vi "ObjectHandler.ExitReference.vi"(8 "error in (no error)":errorcluster, 10 "Name":string, 11 "ObjectHandler in":refnum<class "ObjectHandler.lvclass">) -> (0 "error out":errorcluster, 3 "ObjectHandler out":refnum<class "ObjectHandler.lvclass">)   [LabVIEW 2016, in "ObjectHandler.lvclass"]
uses:
  ObjectHandler.lvclass
  ObjectHandler.ObjectWType.ctl
  ObjectHandler.ObjectType.ctl
  ObjectHandler.lvclass/ObjectHandler.ctl
  ViHandler/ViHandler.lvclass
  Package ErrorHandling/ErrorHandling.lvclass
  CentralStorage/CentralStorage.lvclass
  Package Simulation/Modell/Hausmodell/Hausmodell.lvclass
  Package Simulation/Modell/Sondenmodell/Sondenmodell.lvclass
  Package Simulation/Modell/Umgebung/Umgebung.lvclass
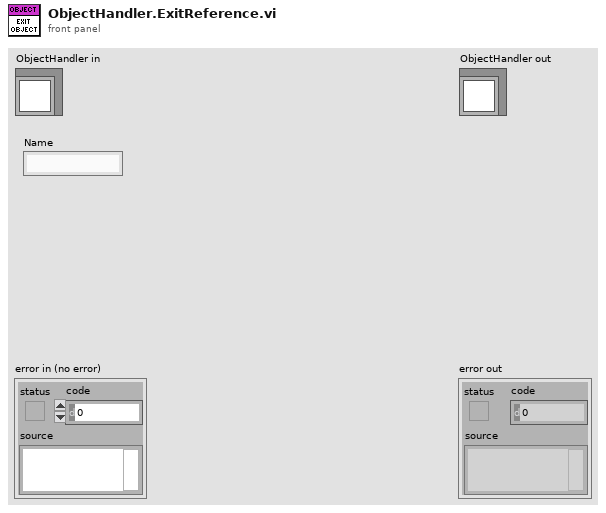
[diagram p1: front panel]
types:
  T1 = typedef "ObjectHandler.lvclass/ObjectHandler.ObjectWType.ctl" = cluster{"ObjectType":T2, "Object":variant}
  T2 = typedef "ObjectHandler.lvclass/ObjectHandler.ObjectType.ctl" = enum16{"undefined", "ObjectHandler", "ViHandler", "ErrorHandler", "CentralStorage", "Hausmodell", "Sondenmodell", "Wärmepumpe", "Umgebung"}
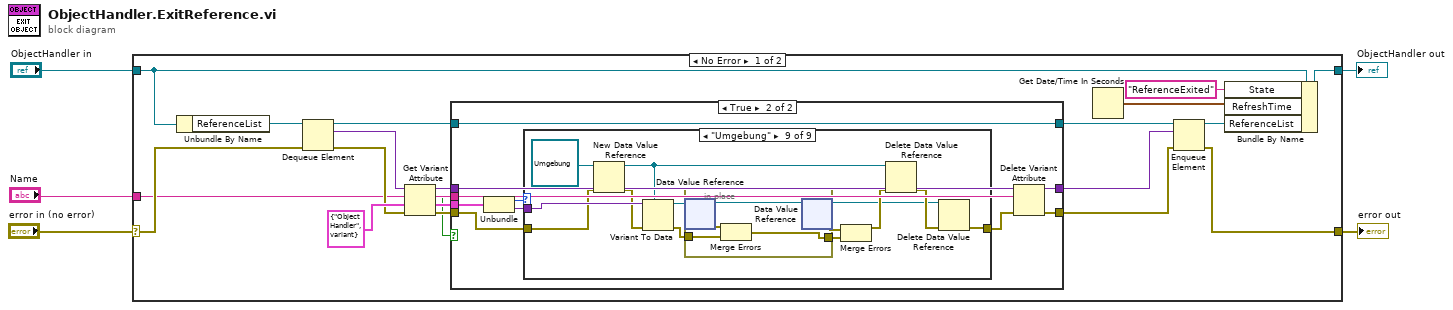
[diagram p0: block diagram]
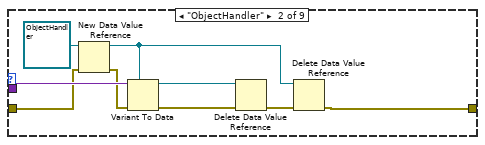
[diagram p4: hidden frame]
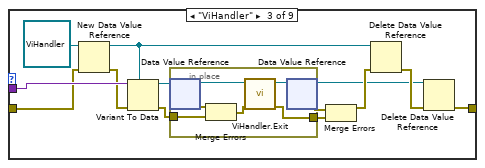
[diagram p5: hidden frame]
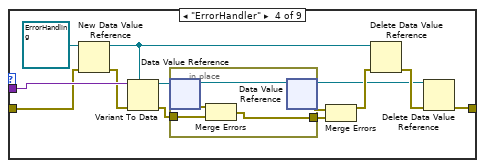
[diagram p6: hidden frame]
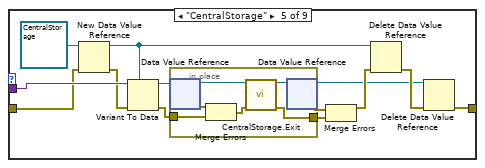
[diagram p7: hidden frame]
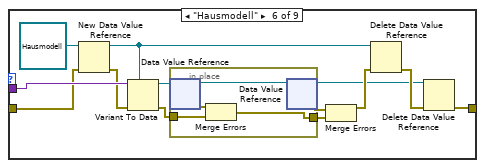
[diagram p8: hidden frame]
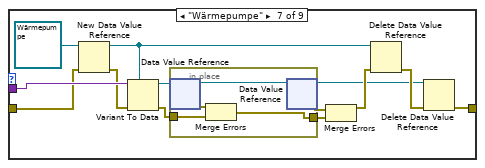
[diagram p9: hidden frame]
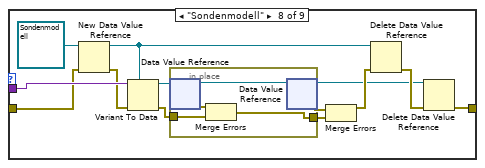
[diagram p10: hidden frame]
diagram:
  n1 = case shown="No Error" "error in (no error)" {
    selector: "error in (no error)" -> [w18 w173]
    tunnel: [w12 w173] -> w4
    tunnel: [w20 w172] -> w2
    tunnel: "ObjectHandler in" -> [w24 w172]
    tunnel: "Name" -> [w9 _]
    frame No Error {
      n2 = Unbundle By Name(w24) -> ("ReferenceList"=w19:refnum<queue>)
      n3 = Dequeue Element(queue=w19, error in (no error)=w18) -> (queue out=w7:refnum<queue>, element=w17:variant, error out=w16:errorcluster)  [unwired: 1 in, 1 out]
      n4 = Get Variant Attribute(Variant=w17, name=w9, default value (empty Variant)=T1 {"ObjectType"=enum."ObjectHandler", "Object"=variant} ("ObjectWType"), error in=w16) -> (duplicate Variant=w21:variant, found=w8:bool, value=w23:T1, error out=w22:errorcluster)
      n5 = case shown="True" w8 {
        tunnel: w23 -> [_ w36]
        tunnel: w22 -> [w28 w35]
        tunnel: w21 -> [w27 w33]
        tunnel: [w27 w32] -> w14
        tunnel: [w28 w31] -> w13
        tunnel: w9 -> [_ w30]
        tunnel: w7 -> [w26 w29]
        tunnel: [w26 w29] -> w6
        frame False {
        }
        frame True {
          n6 = Unbundle(w36) -> ("ObjectType"=w37:T2, "Object"=w38:variant)
          n7 = case shown="\"Umgebung\"" w37 {
            tunnel: w38 -> [_ w47 w61 w80 w97 w116 w133 w150 w167]
            tunnel: w35 -> [w39 w45 w59 w78 w95 w114 w131 w148 w165]
            tunnel: [w39 w40 w56 w75 w92 w111 w128 w145 w162] -> w34
            frame "undefined", Default {
            }
            frame "ObjectHandler" {
              n8 = New Data Value Reference(data value=refnum<class "ObjectHandler.lvclass"> refnum ("ObjectHandler.lvclass"), error in=w45) -> (data value reference=w44:refnum<data-value>, error out=w46:errorcluster)
              n9 = Variant To Data(error in=w46, type=w44, Variant=w47) -> (data=w43:refnum<data-value>, error out=w42:errorcluster)
              n10 = Delete Data Value Reference(data value reference=w43, error in=w42) -> (error out=w41:errorcluster)  [unwired: 1 out]
              n11 = Delete Data Value Reference(data value reference=w44, error in=w41) -> (error out=w40:errorcluster)  [unwired: 1 out]
            }
            frame "ViHandler" {
              n12 = New Data Value Reference(data value=refnum<class "ViHandler.lvclass"> refnum ("ViHandler.lvclass"), error in=w59) -> (data value reference=w58:refnum<data-value>, error out=w60:errorcluster)
              n13 = Variant To Data(error in=w60, type=w58, Variant=w61) -> (data=w55:refnum<data-value>, error out=w54:errorcluster)
              n14 = in-place {
                in-place-border: w54 -> [w66]
                in-place-border: [w62] -> w52
                n15 = in-place-dvr #1(w55) -> (w65:refnum<class "ViHandler.lvclass">, w67:errorcluster)
                n16 = Merge Errors(w67, w66) -> (w63:errorcluster)
                n17 = call "ViHandler.Exit.vi"("error in (no error)"=w63, "ViHandler in"=w65) -> ("error out"=w62:errorcluster, "ViHandler out"=w64:refnum<class "ViHandler.lvclass">)  [unwired: 8 in]
                n18 = in-place-dvr #1(w64) -> (w49:refnum<data-value>, w53:errorcluster)
              }
              n19 = Merge Errors(w53, w52) -> (w51:errorcluster)
              n20 = Delete Data Value Reference(data value reference=w58, error in=w51) -> (error out=w57:errorcluster)  [unwired: 1 out]
              n21 = Delete Data Value Reference(data value reference=w49, error in=w57) -> (error out=w56:errorcluster)  [unwired: 1 out]
            }
            frame "ErrorHandler" {
              n22 = New Data Value Reference(data value=refnum<class "ErrorHandling.lvclass"> refnum ("ErrorHandling.lvclass"), error in=w78) -> (data value reference=w77:refnum<data-value>, error out=w79:errorcluster)
              n23 = Variant To Data(error in=w79, type=w77, Variant=w80) -> (data=w74:refnum<data-value>, error out=w73:errorcluster)
              n24 = in-place {
                in-place-border: w73 -> [w83]
                in-place-border: [w81] -> w71
                n25 = in-place-dvr #2(w74) -> (w82:refnum<class "ErrorHandling.lvclass">, w84:errorcluster)
                n26 = Merge Errors(w84, w83) -> (w81:errorcluster)
                n27 = in-place-dvr #2(w82) -> (w69:refnum<data-value>, w72:errorcluster)
              }
              n28 = Merge Errors(w72, w71) -> (w70:errorcluster)
              n29 = Delete Data Value Reference(data value reference=w77, error in=w70) -> (error out=w76:errorcluster)  [unwired: 1 out]
              n30 = Delete Data Value Reference(data value reference=w69, error in=w76) -> (error out=w75:errorcluster)  [unwired: 1 out]
            }
            frame "CentralStorage" {
              n31 = New Data Value Reference(data value=refnum<class "CentralStorage.lvclass"> refnum ("CentralStorage.lvclass"), error in=w95) -> (data value reference=w94:refnum<data-value>, error out=w96:errorcluster)
              n32 = Variant To Data(error in=w96, type=w94, Variant=w97) -> (data=w91:refnum<data-value>, error out=w90:errorcluster)
              n33 = in-place {
                in-place-border: w90 -> [w102]
                in-place-border: [w98] -> w88
                n34 = in-place-dvr #3(w91) -> (w101:refnum<class "CentralStorage.lvclass">, w103:errorcluster)
                n35 = Merge Errors(w103, w102) -> (w99:errorcluster)
                n36 = call "CentralStorage.Exit.vi"("error in (no error)"=w99, "CentralStorage in"=w101) -> ("error out"=w98:errorcluster, "CentralStorage out"=w100:refnum<class "CentralStorage.lvclass">)  [unwired: 8 in]
                n37 = in-place-dvr #3(w100) -> (w86:refnum<data-value>, w89:errorcluster)
              }
              n38 = Merge Errors(w89, w88) -> (w87:errorcluster)
              n39 = Delete Data Value Reference(data value reference=w94, error in=w87) -> (error out=w93:errorcluster)  [unwired: 1 out]
              n40 = Delete Data Value Reference(data value reference=w86, error in=w93) -> (error out=w92:errorcluster)  [unwired: 1 out]
            }
            frame "Hausmodell" {
              n41 = New Data Value Reference(data value=refnum<class "Hausmodell.lvclass"> refnum ("Hausmodell.lvclass"), error in=w114) -> (data value reference=w113:refnum<data-value>, error out=w115:errorcluster)
              n42 = Variant To Data(error in=w115, type=w113, Variant=w116) -> (data=w110:refnum<data-value>, error out=w109:errorcluster)
              n43 = in-place {
                in-place-border: w109 -> [w119]
                in-place-border: [w117] -> w107
                n44 = in-place-dvr #4(w110) -> (w118:refnum<class "Hausmodell.lvclass">, w120:errorcluster)
                n45 = Merge Errors(w120, w119) -> (w117:errorcluster)
                n46 = in-place-dvr #4(w118) -> (w105:refnum<data-value>, w108:errorcluster)
              }
              n47 = Merge Errors(w108, w107) -> (w106:errorcluster)
              n48 = Delete Data Value Reference(data value reference=w113, error in=w106) -> (error out=w112:errorcluster)  [unwired: 1 out]
              n49 = Delete Data Value Reference(data value reference=w105, error in=w112) -> (error out=w111:errorcluster)  [unwired: 1 out]
            }
            frame "Wärmepumpe" {
              n50 = New Data Value Reference(data value=refnum<class "Wärmepumpe.lvclass"> refnum ("Wärmepumpe.lvclass"), error in=w131) -> (data value reference=w130:refnum<data-value>, error out=w132:errorcluster)
              n51 = Variant To Data(error in=w132, type=w130, Variant=w133) -> (data=w127:refnum<data-value>, error out=w126:errorcluster)
              n52 = in-place {
                in-place-border: w126 -> [w136]
                in-place-border: [w134] -> w124
                n53 = in-place-dvr #5(w127) -> (w135:refnum<class "Wärmepumpe.lvclass">, w137:errorcluster)
                n54 = Merge Errors(w137, w136) -> (w134:errorcluster)
                n55 = in-place-dvr #5(w135) -> (w122:refnum<data-value>, w125:errorcluster)
              }
              n56 = Merge Errors(w125, w124) -> (w123:errorcluster)
              n57 = Delete Data Value Reference(data value reference=w130, error in=w123) -> (error out=w129:errorcluster)  [unwired: 1 out]
              n58 = Delete Data Value Reference(data value reference=w122, error in=w129) -> (error out=w128:errorcluster)  [unwired: 1 out]
            }
            frame "Sondenmodell" {
              n59 = New Data Value Reference(data value=refnum<class "Sondenmodell.lvclass"> refnum ("Sondenmodell.lvclass"), error in=w148) -> (data value reference=w147:refnum<data-value>, error out=w149:errorcluster)
              n60 = Variant To Data(error in=w149, type=w147, Variant=w150) -> (data=w144:refnum<data-value>, error out=w143:errorcluster)
              n61 = in-place {
                in-place-border: w143 -> [w153]
                in-place-border: [w151] -> w141
                n62 = in-place-dvr #6(w144) -> (w152:refnum<class "Sondenmodell.lvclass">, w154:errorcluster)
                n63 = Merge Errors(w154, w153) -> (w151:errorcluster)
                n64 = in-place-dvr #6(w152) -> (w139:refnum<data-value>, w142:errorcluster)
              }
              n65 = Merge Errors(w142, w141) -> (w140:errorcluster)
              n66 = Delete Data Value Reference(data value reference=w147, error in=w140) -> (error out=w146:errorcluster)  [unwired: 1 out]
              n67 = Delete Data Value Reference(data value reference=w139, error in=w146) -> (error out=w145:errorcluster)  [unwired: 1 out]
            }
            frame "Umgebung" {
              n68 = New Data Value Reference(data value=refnum<class "Umgebung.lvclass"> refnum ("Umgebung.lvclass"), error in=w165) -> (data value reference=w164:refnum<data-value>, error out=w166:errorcluster)
              n69 = Variant To Data(error in=w166, type=w164, Variant=w167) -> (data=w161:refnum<data-value>, error out=w160:errorcluster)
              n70 = in-place {
                in-place-border: w160 -> [w170]
                in-place-border: [w168] -> w158
                n71 = in-place-dvr #7(w161) -> (w169:refnum<class "Umgebung.lvclass">, w171:errorcluster)
                n72 = Merge Errors(w171, w170) -> (w168:errorcluster)
                n73 = in-place-dvr #7(w169) -> (w156:refnum<data-value>, w159:errorcluster)
              }
              n74 = Merge Errors(w159, w158) -> (w157:errorcluster)
              n75 = Delete Data Value Reference(data value reference=w164, error in=w157) -> (error out=w163:errorcluster)  [unwired: 1 out]
              n76 = Delete Data Value Reference(data value reference=w156, error in=w163) -> (error out=w162:errorcluster)  [unwired: 1 out]
            }
          }
          n77 = Delete Variant Attribute(4:w34, 6:w30, 7:w33) -> (0:w31:errorcluster, 3:w32:variant)  [unwired: 1 out]
        }
      }
      n78 = Get Date/Time In Seconds() -> (seconds since 1Jan1904=w10:timestamp)
      n79 = Enqueue Element(queue=w6, element=w14, error in (no error)=w13) -> (queue out=w15:refnum<queue>, error out=w12:errorcluster)  [unwired: 1 in, 1 out]
      n80 = Bundle By Name(cluster=w24, "State"="ReferenceExited", "RefreshTime"=w10, "ReferenceList"=w15) -> (w20:refnum<class "ObjectHandler.lvclass">)
    }
    frame Error {
    }
  }
  "error out" <- w4
  "ObjectHandler out" <- w2
